vi "multiplexor_main_v19.0.vi"() -> ()   [LabVIEW 2019]
uses:
  <vilib>/Instr/_visa.llb/VISA Configure Serial Port (Instr).vi
panel:
  in  "Tension":string(combo)
  in  "Corriente":string(combo)
  out "COMMAND":string
  in  "Lock-In B":string(combo)
  in  "Lock-In A":string(combo)
  in  "Arb command 2":bool
  out "Boolean 14":bool
  out "Boolean 13":bool
  out "Boolean 12":bool
  out "Boolean 11":bool
  out "Boolean 10":bool
  out "Boolean 9":bool
  out "Boolean 8":bool
  out "Boolean 7":bool
  out "Boolean 6":bool
  out "Boolean 5":bool
  out "Boolean 4":bool
  out "Boolean 3":bool
  in  "ARB COMMAND":string="1"
  in  "Arb command":bool
  in  "RST":bool
  in  "M2":bool
  in  "M3":bool
  in  "R/L":bool
  in  "M1":bool
  in  "SGs":bool
  in  "VISA resource name":refnum<visa-resource-name>
  # "MULTIPLEXOR"
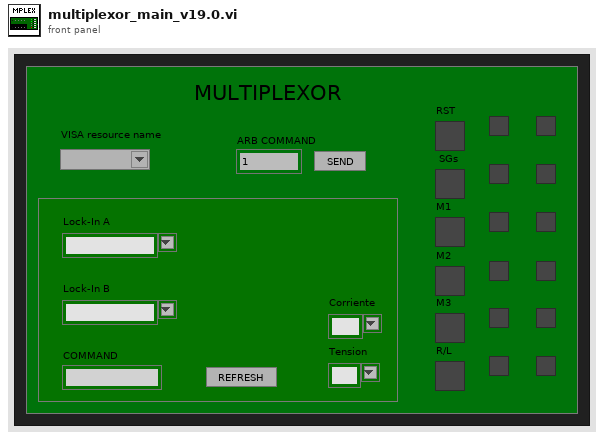
[diagram p1: front panel]
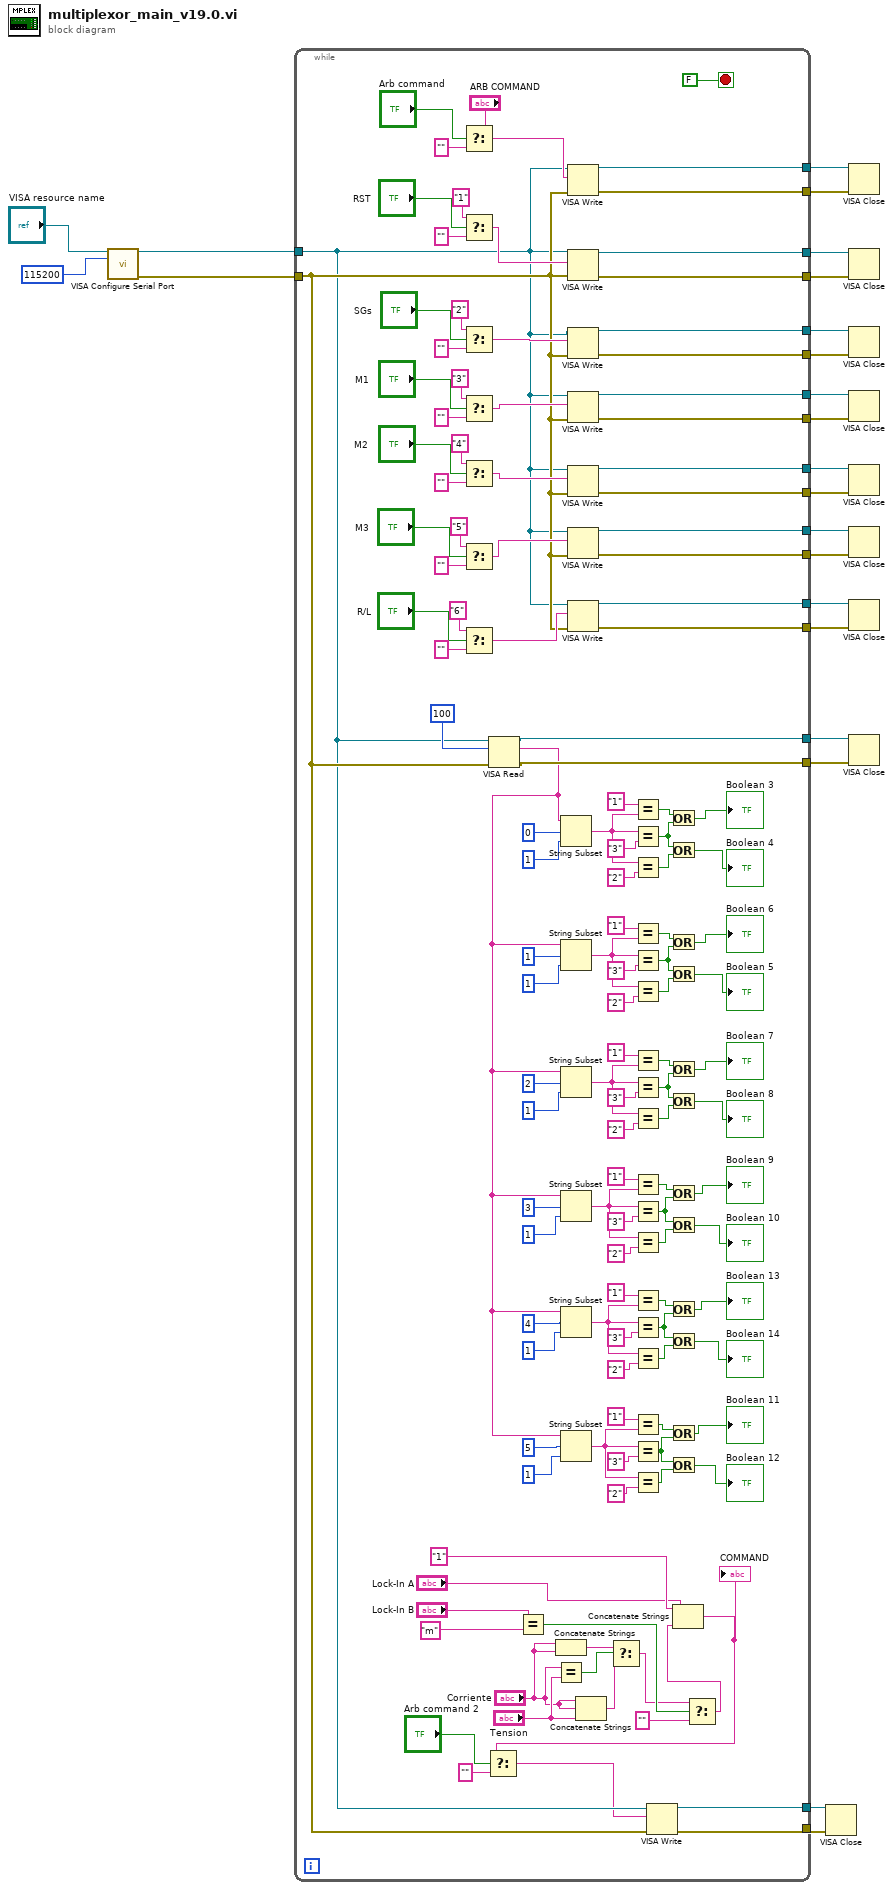
[diagram p0: block diagram]
diagram:
  n1 = call-poly "VISA Configure Serial Port"("VISA resource name"="VISA resource name", "baud rate (9600)"=u32 115200) -> ("VISA resource name out"=w22:refnum<visa-resource-name>, "error out"=w20:errorcluster)  [unwired: 12 in]
  n2 = while {
    tunnel: w22 -> [w40]
    tunnel: [w156] -> w21
    tunnel: w20 -> [w41]
    tunnel: [w155] -> w19
    tunnel: [w153] -> w16
    tunnel: [w154] -> w17
    tunnel: [w152] -> w15
    tunnel: [w151] -> w14
    tunnel: [w149] -> w12
    tunnel: [w150] -> w13
    tunnel: [w148] -> w11
    tunnel: [w147] -> w10
    tunnel: [w145] -> w8
    tunnel: [w146] -> w9
    tunnel: [w118] -> w5
    tunnel: [w119] -> w6
    tunnel: [w113] -> w4
    tunnel: [w112] -> w3
    tunnel: [w38] -> w2
    tunnel: [w37] -> w1
    stop <- FALSE stop-if-true
    n3 = Select(t="ARB COMMAND", s="Arb command", f="") -> (s? t:f=w114:string)
    n4 = Select(t="1" ("write buffer"), s="RST", f="") -> (s? t:f=w121:string)
    n5 = Select(t="2" ("write buffer"), s="SGs", f="") -> (s? t:f=w120:string)
    n6 = Select(t="3" ("write buffer"), s="M1", f="") -> (s? t:f=w128:string)
    n7 = Select(t="4" ("write buffer"), s="M2", f="") -> (s? t:f=w127:string)
    n8 = Select(t="5" ("write buffer"), s="M3", f="") -> (s? t:f=w126:string)
    n9 = Select(t="6" ("write buffer"), s="R/L", f="") -> (s? t:f=w125:string)
    n10 = VISA Read(VISA resource name=w40, byte count=u32 100, error in (no error)=w41) -> (VISA resource name out=w112:refnum<visa-resource-name>, read buffer=w46:string, error out=w113:errorcluster)  [unwired: 1 out]
    n11 = Equal?(x="Lock-In B", y="m") -> (x = y?=w31:bool)
    n12 = Concatenate Strings("Corriente", "Corriente") -> (w23:string)
    n13 = Equal?(x="Corriente", y="Tension") -> (x = y?=w28:bool)
    n14 = String Subset(string=w46, offset (0)=0, length (rest)=1 ("length (rest)")) -> (substring=w100:string)
    n15 = String Subset(string=w46, offset (0)=1, length (rest)=1 ("length (rest)")) -> (substring=w45:string)
    n16 = String Subset(string=w46, offset (0)=2, length (rest)=1 ("length (rest)")) -> (substring=w44:string)
    n17 = String Subset(string=w46, offset (0)=3, length (rest)=1 ("length (rest)")) -> (substring=w69:string)
    n18 = String Subset(string=w46, offset (0)=4, length (rest)=1 ("length (rest)")) -> (substring=w47:string)
    n19 = String Subset(string=w46, offset (0)=5, length (rest)=1 ("length (rest)")) -> (substring=w68:string)
    n20 = VISA Write(VISA resource name=w40, write buffer=w114, error in (no error)=w41) -> (VISA resource name out=w118:refnum<visa-resource-name>, error out=w119:errorcluster)  [unwired: 1 out]
    n21 = VISA Write(VISA resource name=w40, write buffer=w121, error in (no error)=w41) -> (VISA resource name out=w156:refnum<visa-resource-name>, error out=w155:errorcluster)  [unwired: 1 out]
    n22 = VISA Write(VISA resource name=w40, write buffer=w120, error in (no error)=w41) -> (VISA resource name out=w153:refnum<visa-resource-name>, error out=w154:errorcluster)  [unwired: 1 out]
    n23 = VISA Write(VISA resource name=w40, write buffer=w128, error in (no error)=w41) -> (VISA resource name out=w152:refnum<visa-resource-name>, error out=w151:errorcluster)  [unwired: 1 out]
    n24 = VISA Write(VISA resource name=w40, write buffer=w127, error in (no error)=w41) -> (VISA resource name out=w149:refnum<visa-resource-name>, error out=w150:errorcluster)  [unwired: 1 out]
    n25 = VISA Write(VISA resource name=w40, write buffer=w126, error in (no error)=w41) -> (VISA resource name out=w148:refnum<visa-resource-name>, error out=w147:errorcluster)  [unwired: 1 out]
    n26 = VISA Write(VISA resource name=w40, write buffer=w125, error in (no error)=w41) -> (VISA resource name out=w145:refnum<visa-resource-name>, error out=w146:errorcluster)  [unwired: 1 out]
    n27 = Concatenate Strings("Corriente", "Corriente", "Tension") -> (w26:string)
    n28 = Select(t=w23, s=w28, f=w26) -> (s? t:f=w25:string)
    n29 = Equal?(x="1", y=w100) -> (x = y?=w106:bool)
    n30 = Equal?(x=w100, y="3") -> (x = y?=w108:bool)
    n31 = Equal?(x=w100, y="2") -> (x = y?=w107:bool)
    n32 = Equal?(x="1", y=w45) -> (x = y?=w95:bool)
    n33 = Equal?(x=w45, y="3") -> (x = y?=w97:bool)
    n34 = Equal?(x=w45, y="2") -> (x = y?=w96:bool)
    n35 = Equal?(x="1", y=w44) -> (x = y?=w84:bool)
    n36 = Equal?(x=w44, y="3") -> (x = y?=w82:bool)
    n37 = Equal?(x=w44, y="2") -> (x = y?=w83:bool)
    n38 = Equal?(x="1", y=w69) -> (x = y?=w75:bool)
    n39 = Equal?(x=w69, y="3") -> (x = y?=w77:bool)
    n40 = Equal?(x=w69, y="2") -> (x = y?=w76:bool)
    n41 = Equal?(x="1", y=w47) -> (x = y?=w53:bool)
    n42 = Equal?(x=w47, y="3") -> (x = y?=w55:bool)
    n43 = Equal?(x=w47, y="2") -> (x = y?=w54:bool)
    n44 = Equal?(x="1", y=w68) -> (x = y?=w62:bool)
    n45 = Equal?(x=w68, y="3") -> (x = y?=w60:bool)
    n46 = Equal?(x=w68, y="2") -> (x = y?=w61:bool)
    n47 = Or(x=w106, y=w108) -> (x .or. y?=→"Boolean 3":bool)
    n48 = Or(x=w108, y=w107) -> (x .or. y?=→"Boolean 4":bool)
    n49 = Or(x=w95, y=w97) -> (x .or. y?=→"Boolean 6":bool)
    n50 = Or(x=w97, y=w96) -> (x .or. y?=→"Boolean 5":bool)
    n51 = Or(x=w84, y=w82) -> (x .or. y?=→"Boolean 7":bool)
    n52 = Or(x=w82, y=w83) -> (x .or. y?=→"Boolean 8":bool)
    n53 = Or(x=w75, y=w77) -> (x .or. y?=→"Boolean 9":bool)
    n54 = Or(x=w77, y=w76) -> (x .or. y?=→"Boolean 10":bool)
    n55 = Or(x=w53, y=w55) -> (x .or. y?=→"Boolean 13":bool)
    n56 = Or(x=w55, y=w54) -> (x .or. y?=→"Boolean 14":bool)
    n57 = Or(x=w62, y=w60) -> (x .or. y?=→"Boolean 11":bool)
    n58 = Or(x=w60, y=w61) -> (x .or. y?=→"Boolean 12":bool)
    n59 = Select(t=w25, s=w31, f="") -> (s? t:f=w29:string)
    n60 = Concatenate Strings("1" ("string"), "Lock-In A", w29) -> (w30:string)
    "COMMAND" <- w30
    n61 = Select(t=w30, s="Arb command 2", f="") -> (s? t:f=w39:string)
    n62 = VISA Write(VISA resource name=w40, write buffer=w39, error in (no error)=w41) -> (VISA resource name out=w37:refnum<visa-resource-name>, error out=w38:errorcluster)  [unwired: 1 out]
  }
  n63 = VISA Close(VISA resource name=w1, error in (no error)=w2) -> ()  [unwired: 1 out]
  n64 = VISA Close(VISA resource name=w5, error in (no error)=w6) -> ()  [unwired: 1 out]
  n65 = VISA Close(VISA resource name=w21, error in (no error)=w19) -> ()  [unwired: 1 out]
  n66 = VISA Close(VISA resource name=w16, error in (no error)=w17) -> ()  [unwired: 1 out]
  n67 = VISA Close(VISA resource name=w15, error in (no error)=w14) -> ()  [unwired: 1 out]
  n68 = VISA Close(VISA resource name=w12, error in (no error)=w13) -> ()  [unwired: 1 out]
  n69 = VISA Close(VISA resource name=w11, error in (no error)=w10) -> ()  [unwired: 1 out]
  n70 = VISA Close(VISA resource name=w8, error in (no error)=w9) -> ()  [unwired: 1 out]
  n71 = VISA Close(VISA resource name=w3, error in (no error)=w4) -> ()  [unwired: 1 out]
